vi "Configure Load to Single-Ganged.vi"(8 "error in":errorcluster, 10 "measurement configuration":T6 {"Measurement timeout" format="%.3p"; "Load device voltage/current rating" format="%#_6pA"; "Load output function" items=["DC Voltage"=1006, "DC Current"=1007, "Pulse Voltage"=1049, "Pulse Current"=1050]; "Power ON/Source output function" items=["DC Voltage"=1006, "DC Current"=1007, "Pulse Voltage"=1049, "Pulse Current"=1050]; "Load sense" items=["Local"=1008, "Remote"=1009]; "Load transient response" items=["Slow"=1041, "Normal"=1038, "Fast"=1039, "Custom"=1042]; "Power ON/Source sense" items=["Local"=1008, "Remote"=1009]; "Source transient response" items=["Slow"=1041, "Normal"=1038, "Fast"=1039, "Custom"=1042]; "Measurement duration" format="%.3p"; "Aperture time" format="%.3p"; "Load current/voltage limit high" format="%#_6p"; "Load current/voltage limit low" format="%#_6p"; "Load current/voltage limit range" format="%#_6p"; "Load voltage/current level range" format="%#_6p"; "Load voltage/current level" format="%#_6p"; "Source current/voltage limit high" format="%#_6p"; "Source current/voltage limit low" format="%#_6p"; "Power ON/Source current/voltage limit range" format="%#_6p"; "Source voltage/current level range" format="%#_6p"; "Power ON/Source voltage/current level" format="%#_6p"}, 11 "Single Point Perform Measurement in":T1) -> (0 "error out":errorcluster, 3 "Single Point Perform Measurement out":T1)   [LabVIEW 2021, in "Single Point_Channel Ganging.lvlib"]
uses:
  Single Point_Channel Ganging.lvlib
  Measurement Configuration.ctl
  Controls/Perform measurement-control.ctl
  shared subVIs/ctl/NIDCPower_channel_ganging - ctl - ganged session.ctl
  shared subVIs/ctl/NIDCPower_channel_ganging - ctl - ganged config.ctl
  shared subVIs/ctl/NIDCPower_channel_ganging - ctl - channel mode.ctl
  Measurement Results.ctl
  <instrlib>/niDCPower/nidcpower.llb/niDCPower Source Mode.ctl
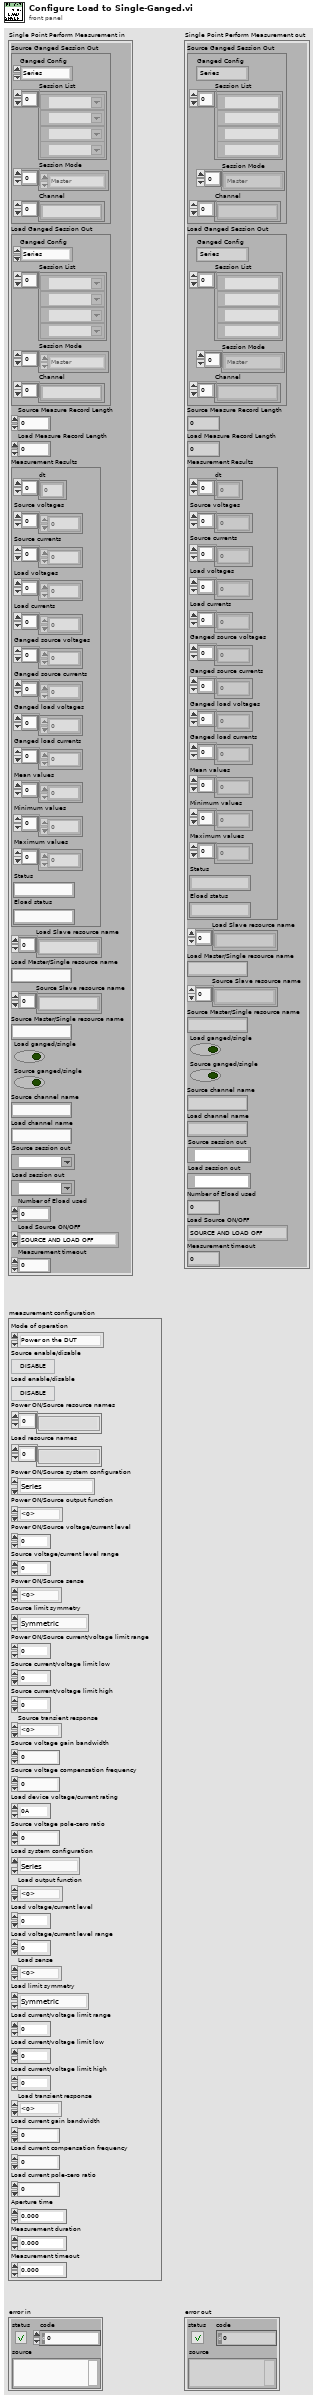
[diagram p1: front panel]
types:
  T1 = typedef "Single Point_Channel Ganging.lvlib/Perform measurement-control.ctl" = cluster{"Source Ganged Session Out":T2, "Load Ganged Session Out":T2, "Source Measure Record Length":i32, "Load Measure Record Length":i32, "Measurement Results":T5, "Load Slave resource name":string[], "Load Master/Single resource name":string, "Source Slave resource name":string[], "Source Master/Single resource name":string, "Load ganged/single":bool, "Source ganged/single":bool, "Source channel name":string, "Load channel name":string, "Source session out":refnum<k15>, "Load session out":refnum<k15>, "Number of Eload used":i32, "Load Source ON/OFF":enum16{"SOURCE AND LOAD OFF", "SOURCE ON", "LOAD ON", "SOURCE AND LOAD ON"}, "Measurement timeout":dbl}
  T2 = typedef "NIDCPower_channel_ganging - ctl - ganged session.ctl" = cluster{"Ganged Config":T3, "Session List":refnum<k15>[], "Session Mode":T4[], "Channel":string[]}
  T3 = typedef "NIDCPower_channel_ganging - ctl - ganged config.ctl" = enum32{"Series", "Parallel", "Manual"}
  T4 = typedef "NIDCPower_channel_ganging - ctl - channel mode.ctl" = enum32{"Master", "Slave", "Slave - Inverted"}
  T5 = typedef "Single Point_Channel Ganging.lvlib/Measurement Results.ctl" = cluster{"dt":dbl[], "Source voltages":dbl[], "Source currents":dbl[], "Load voltages":dbl[], "Load currents":dbl[], "Ganged source voltages":dbl[], "Ganged source currents":dbl[], "Ganged load voltages":dbl[], "Ganged load currents":dbl[], "Mean values":dbl[], "Minimum values":dbl[], "Maximum values":dbl[], "Status":string, "Eload status":string}
  T6 = typedef "Single Point_Channel Ganging.lvlib/Measurement Configuration.ctl" = cluster{"Mode of operation":enum32{"Power on the DUT", "Perform measurement", "Power off the DUT"}, "Source enable/disable":bool, "Load enable/disable":bool, "Power ON/Source resource names":string[], "Load resource names":string[], "Power ON/Source system configuration":enum32{"Series", "Parallel", "Manual"}, "Power ON/Source output function":i32, "Power ON/Source voltage/current level":dbl, "Source voltage/current level range":dbl, "Power ON/Source sense":i32, "Source limit symmetry":enum32{"Symmetric", "Asymmetric"}, "Power ON/Source current/voltage limit range":dbl, "Source current/voltage limit low":dbl, "Source current/voltage limit high":dbl, "Source transient response":i32, "Source voltage gain bandwidth":dbl, "Source voltage compensation frequency":dbl, "Load device voltage/current rating":dbl, "Source voltage pole-zero ratio":dbl, "Load system configuration":enum32{"Series", "Parallel", "Manual"}, "Load output function":i32, "Load voltage/current level":dbl, "Load voltage/current level range":dbl, "Load sense":i32, "Load limit symmetry":enum32{"Symmetric", "Asymmetric"}, "Load current/voltage limit range":dbl, "Load current/voltage limit low":dbl, "Load current/voltage limit high":dbl, "Load transient response":i32, "Load current gain bandwidth":dbl, "Load current compensation frequency":dbl, "Load current pole-zero ratio":dbl, "Aperture time":dbl, "Measurement duration":dbl, "Measurement timeout":dbl}
  T7 = typedef "niDCPower Source Mode.ctl" = i32
  T8 = typedef "NIDCPower_channel_ganging - ctl - channel def.ctl" = cluster{"resource name":refnum<k15>, "channels":string, "Channel Mode":T4}
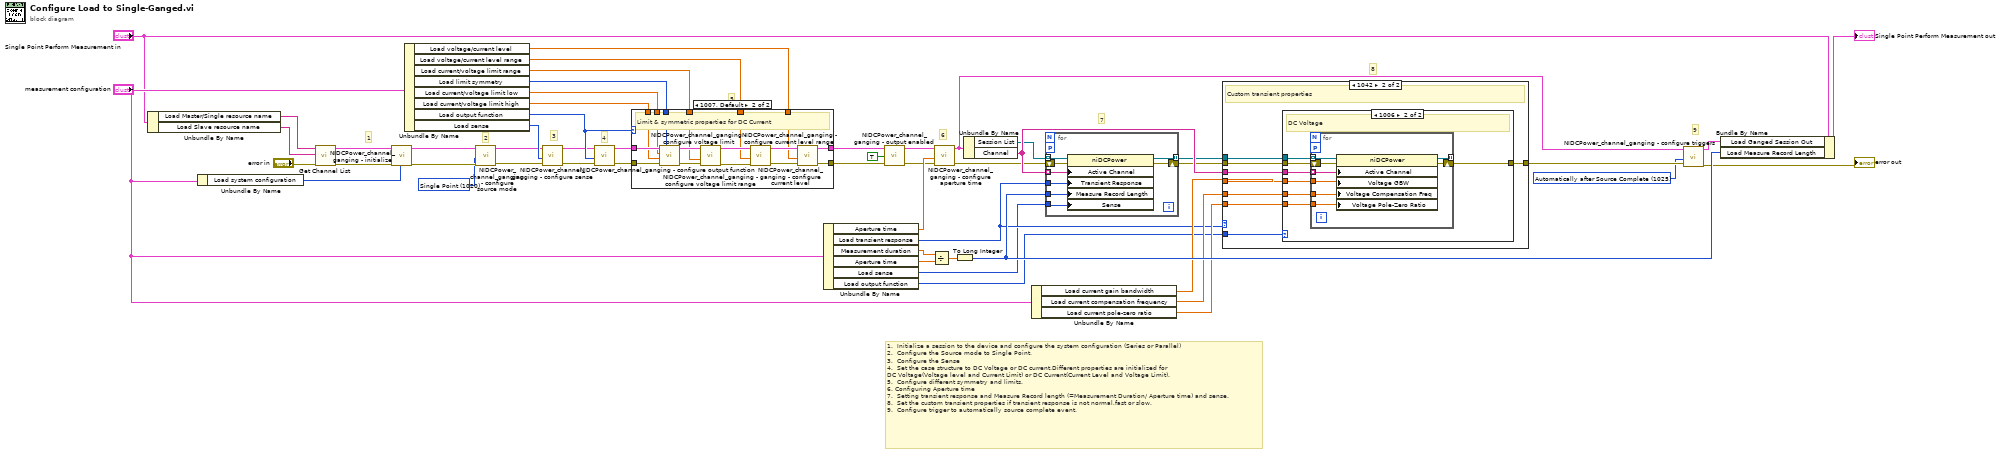
[diagram p0: block diagram]
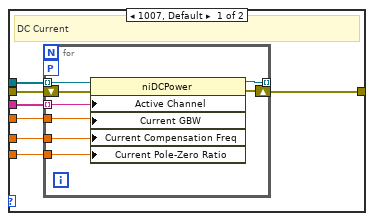
[diagram p3: hidden frame]
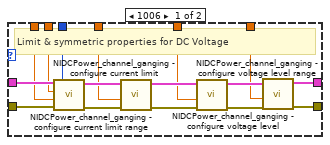
[diagram p4: hidden frame]
diagram:
  w34 = 1025 items=["Automatically after Source Complete"=1025, "On Demand"=1026, "On Measure Trigger"=1027] ("Measure When")
  w1 = T7 1020 items=["Single Point"=1020, "Sequence"=1021] ("source mode")
  # "4"
  # "3"
  # "2"
  # "1"
  # "5"
  # "6"
  # "7"
  # "8"
  # "9"
  # "1.  Initialize a session to the device and configure the system configuration (Series or Parallel)\n2.  Configure the Source mode to Single Point.\n3.  Configure the Sense\n4.  Set the case structure to DC Voltage or DC current.Different properties are initialized for \nDC Voltage(Voltage level and Current Limit) or DC Current(Current Level and Voltage Limit). \n5.  Configure different symmetry and limits.\n6. Configuring Aperture time\n7.  Setting transient response and Measure Record length (=Measurement Duration/ Aperture time) and sense.\n8.  Set the custom transient properties if transient response is not normal,fast or slow.\n9.  Configure trigger to automatically source complete event."
  n1 = Unbundle By Name("Single Point Perform Measurement in") -> ("Load Master/Single resource name"=w23:string, "Load Slave resource name"=w24:string[])
  n2 = Unbundle By Name("measurement configuration") -> ("Load system configuration"=w47:enum32{"Series", "Parallel", "Manual"})
  n3 = call "Get Channel List.vi"("error in (no error)"="error in", "Slave resource names"=w24, "Master resouce name"=w23) -> ("error out"=w26:errorcluster, "Channel List"=w25:T8[])  [unwired: 7 in]
  n4 = call "NIDCPower_channel_ganging - initialize.vi"("Ganged Config"=w47, "error in (no error)"=w26, "Channel List"=w25) -> ("error out"=w2:errorcluster, "Ganged Session Out"=w3:T2)  [unwired: 7 in]
  n5 = Unbundle By Name("measurement configuration") -> ("Load voltage/current level"=w18:dbl, "Load voltage/current level range"=w17:dbl, "Load current/voltage limit range"=w16:dbl, "Load limit symmetry"=w15:enum32{"Symmetric", "Asymmetric"}, "Load current/voltage limit low"=w14:dbl, "Load current/voltage limit high"=w13:dbl, "Load output function"=w21:i32, "Load sense"=w20:i32)
  n6 = call "NIDCPower_channel_ganging - configure source mode.vi"("error in (no error)"=w2, "source mode"=w1, "Ganged Session In"=w3) -> ("error out"=w8:errorcluster, "Ganged Session Out"=w7:T2)  [unwired: 7 in]
  n7 = call "NIDCPower_channel_ganging - configure sense.vi"("error in (no error)"=w8, "sense"=w20, "Ganged Session In"=w7) -> ("error out"=w10:errorcluster, "Ganged Session Out"=w9:T2)  [unwired: 7 in]
  n8 = call "NIDCPower_channel_ganging - configure output function.vi"("error in (no error)"=w10, "output function"=w21, "Ganged Session In"=w9) -> ("error out"=w5:errorcluster, "Ganged Session Out"=w4:T2)  [unwired: 7 in]
  n9 = case shown="1007, Default" w21 {
    tunnel: w4 -> [w62 w84]
    tunnel: w5 -> [w66 w83]
    tunnel: w15 -> [w56 w69]
    tunnel: w14 -> [w57 w70]
    tunnel: w13 -> [w58 w74]
    tunnel: w16 -> [w55 w72]
    tunnel: w17 -> [w54 w73]
    tunnel: [w68 w76] -> w11
    tunnel: [w67 w75] -> w12
    tunnel: w18 -> [w53 w71]
    frame 1006 {
      # "Limit & symmetric properties for DC Voltage"
      n10 = call "NIDCPower_channel_ganging - configure current limit.vi"("Limit Symmetry"=w56, "error in (no error)"=w66, "Current limit/hi"=w58, "Current limit lo"=w57, "Ganged Session In"=w62) -> ("error out"=w65:errorcluster, "Ganged Session Out"=w61:T2)  [unwired: 5 in]
      n11 = call "NIDCPower_channel_ganging - configure current limit range.vi"("error in (no error)"=w65, "current limit range"=w55, "Ganged Session In"=w61) -> ("error out"=w64:errorcluster, "Ganged Session Out"=w60:T2)  [unwired: 7 in]
      n12 = call "NIDCPower_channel_ganging - configure voltage level range.vi"("error in (no error)"=w64, "voltage level range"=w54, "Ganged Session In"=w60) -> ("error out"=w63:errorcluster, "Ganged Session Out"=w59:T2)  [unwired: 7 in]
      n13 = call "NIDCPower_channel_ganging - configure voltage level.vi"("error in (no error)"=w63, "voltage level"=w53, "Ganged Session In"=w59) -> ("error out"=w68:errorcluster, "Ganged Session Out"=w67:T2)  [unwired: 7 in]
    }
    frame 1007, Default {
      # "Limit & symmetric properties for DC Current"
      n14 = call "NIDCPower_channel_ganging - configure voltage limit.vi"("Limit Symmetry"=w69, "error in (no error)"=w83, "voltage limit/hi"=w74, "voltage limit lo"=w70, "Ganged Session In"=w84) -> ("error out"=w81:errorcluster, "Ganged Session Out"=w82:T2)  [unwired: 5 in]
      n15 = call "NIDCPower_channel_ganging - configure voltage limit range.vi"("error in (no error)"=w81, "voltage level range"=w72, "Ganged Session In"=w82) -> ("error out"=w79:errorcluster, "Ganged Session Out"=w80:T2)  [unwired: 7 in]
      n16 = call "NIDCPower_channel_ganging - configure current level range.vi"("error in (no error)"=w79, "current level range"=w73, "Ganged Session In"=w80) -> ("error out"=w77:errorcluster, "Ganged Session Out"=w78:T2)  [unwired: 7 in]
      n17 = call "NIDCPower_channel_ganging - configure current level.vi"("error in (no error)"=w77, "current level"=w71, "Ganged Session In"=w78) -> ("error out"=w76:errorcluster, "Ganged Session Out"=w75:T2)  [unwired: 7 in]
    }
  }
  n18 = Unbundle By Name("measurement configuration") -> ("Aperture time"=w52:dbl, "Load transient response"=w38:i32, "Measurement duration"=w36:dbl, "Aperture time"=w51:dbl, "Load sense"=w33:i32, "Load output function"=w37:i32)
  n19 = call "NIDCPower_channel_ganging - output enabled.vi"("error in (no error)"=w11, "output enabled"=TRUE, "Ganged Session In"=w12) -> ("error out"=w30:errorcluster, "Ganged Session Out"=w29:T2)  [unwired: 7 in]
  n20 = Divide(x=w36, y=w51) -> (x/y=w35:dbl)
  n21 = call "NIDCPower_channel_ganging - configure aperture time.vi"("error in (no error)"=w30, "aperture time"=w52, "Ganged Session In"=w29) -> ("error out"=w31:errorcluster, "Ganged Session Out"=w43:T2)  [unwired: 7 in]
  n22 = To Long Integer(number=w35) -> (32bit integer=w50:i32)
  n23 = Unbundle By Name(w43) -> ("Session List"=w32:refnum<k15>[], "Channel"=w42:string[])
  n24 = Unbundle By Name("measurement configuration") -> ("Load current gain bandwidth"=w44:dbl, "Load current compensation frequency"=w45:dbl, "Load current pole-zero ratio"=w46:dbl)
  n25 = for {
    tunnel: [w92] -> w39 mode=indexing
    shift-right: [w90] -> w40
    shift-left: w31 -> [w91]
    workers-P: _ -> [_]
    tunnel: w32 -> [w89] mode=indexing
    tunnel: w33 -> [w88]
    tunnel: w38 -> [w86]
    tunnel: w50 -> [w87]
    tunnel: w42 -> [w85] mode=indexing
    n26 = property class="niDCPower"(reference=w89, error in=w91, "Active Channel"=w85, "Transient Response"=w86, "Measure Record Length"=w87, "Sense"=w88) -> (reference out=w92:refnum<k15>, error out=w90:errorcluster)
  }
  n27 = case shown="1042" w38 {
    tunnel: w37 -> [_ w101]
    tunnel: w39 -> [_ w100]
    tunnel: w40 -> [w93 w99]
    tunnel: [w93 w98] -> w41
    tunnel: w42 -> [_ w97]
    tunnel: w44 -> [_ w96]
    tunnel: w45 -> [_ w95]
    tunnel: w46 -> [_ w94]
    frame Default {
      # "Normal, slow and fast transient"
    }
    frame 1042 {
      # "Custom transient properties"
      n28 = case shown="1006" w101 {
        tunnel: w99 -> [w108 w123]
        tunnel: [w107 w122] -> w98
        tunnel: w100 -> [w106 w121]
        tunnel: w97 -> [w104 w120]
        tunnel: w96 -> [w105 w119]
        tunnel: w94 -> [w102 w117]
        tunnel: w95 -> [w103 w118]
        frame 1007, Default {
          # "DC Current"
          n29 = for {
            workers-P: _ -> [_]
            shift-right: [w115] -> w107
            shift-left: w108 -> [w116]
            tunnel: w106 -> [w114] mode=indexing
            tunnel: [w113] -> _ mode=indexing
            tunnel: w105 -> [w112]
            tunnel: w104 -> [w111] mode=indexing
            tunnel: w103 -> [w110]
            tunnel: w102 -> [w109]
            n30 = property class="niDCPower"(reference=w114, error in=w116, "Active Channel"=w111, "Current GBW"=w112, "Current Compensation Freq"=w110, "Current Pole-Zero Ratio"=w109) -> (reference out=w113:refnum<k15>, error out=w115:errorcluster)
          }
        }
        frame 1006 {
          # "DC Voltage"
          n31 = for {
            workers-P: _ -> [_]
            shift-right: [w124] -> w122
            shift-left: w123 -> [w131]
            tunnel: w121 -> [w130] mode=indexing
            tunnel: [w129] -> _ mode=indexing
            tunnel: w120 -> [w128] mode=indexing
            tunnel: w119 -> [w127]
            tunnel: w118 -> [w126]
            tunnel: w117 -> [w125]
            n32 = property class="niDCPower"(reference=w130, error in=w131, "Active Channel"=w128, "Voltage GBW"=w127, "Voltage Compensation Freq"=w126, "Voltage Pole-Zero Ratio"=w125) -> (reference out=w129:refnum<k15>, error out=w124:errorcluster)
          }
        }
      }
    }
  }
  n33 = call "NIDCPower_channel_ganging - configure triggers.vi"("error in (no error)"=w41, "Measure When"=w34, "Ganged Session In"=w43) -> ("error out"=→"error out":errorcluster, "Ganged Session Out"=w28:T2)  [unwired: 7 in]
  n34 = Bundle By Name(cluster="Single Point Perform Measurement in", "Load Ganged Session Out"=w28, "Load Measure Record Length"=w50) -> (→"Single Point Perform Measurement out":T1)
